vi "subvi voltage to temp to write.vi"(9 "Thermistor 2":T1={"sampling freq: fs 2"=200.0, "low cutoff freq: fl 2"=5.0, "order 2"=3} {"low cutoff freq: fl 2" format="%#_13g"; "sampling freq: fs 2" format="%#_13g"}, 10 "Thermistor 1":T2, 11 "data":dynamicdata(waveform)) -> (0 "Thermistor 1 and 2":cluster{"Filtered x":dbl, "Filtered x":dbl}(graph))   [LabVIEW 2021]
uses:
  <vilib>/express/express shared/ex_Modify Signal Name.vi
  <vilib>/express/express arith-compare/Formula/XNode/ExpressFormulaBlockNode.xnode
  <vilib>/ptbypt/NI_PtbyPt.lvlib
panel:
  out "Thermistor 2 Filtered":dbl(graph)
  out "Thermistor 2 Unfiltered":waveform(dbl)(graph)
  out "Thermistor 1 Filtered":dbl(graph)
  out "Thermistor 1 Unfiltered":waveform(dbl)(graph)
  out "Waveform Chart":dynamicdata(graph)
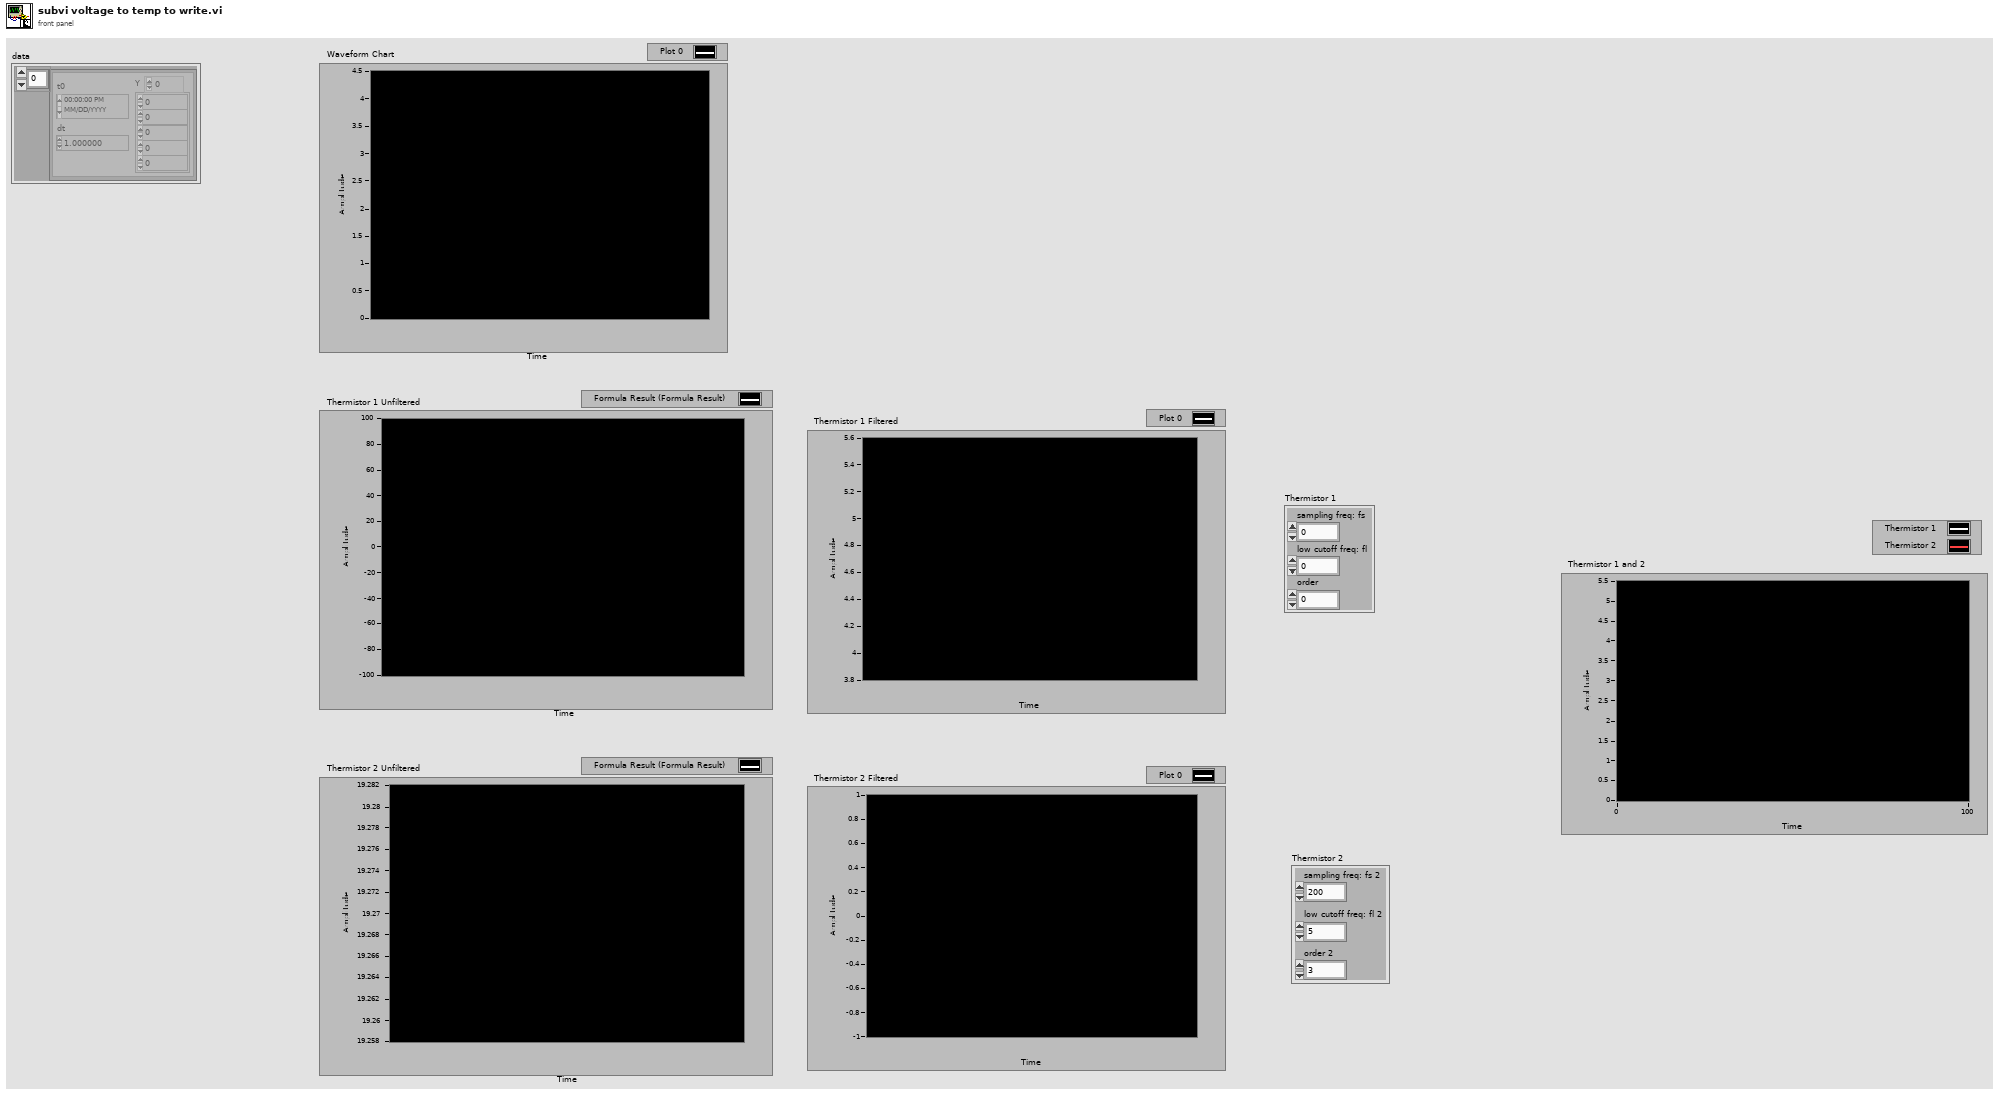
[diagram p1: front panel]
types:
  T1 = cluster{"sampling freq: fs 2":dbl, "low cutoff freq: fl 2":dbl, "order 2":i32}
  T2 = cluster{"sampling freq: fs":dbl, "low cutoff freq: fl":dbl, "order":i32}
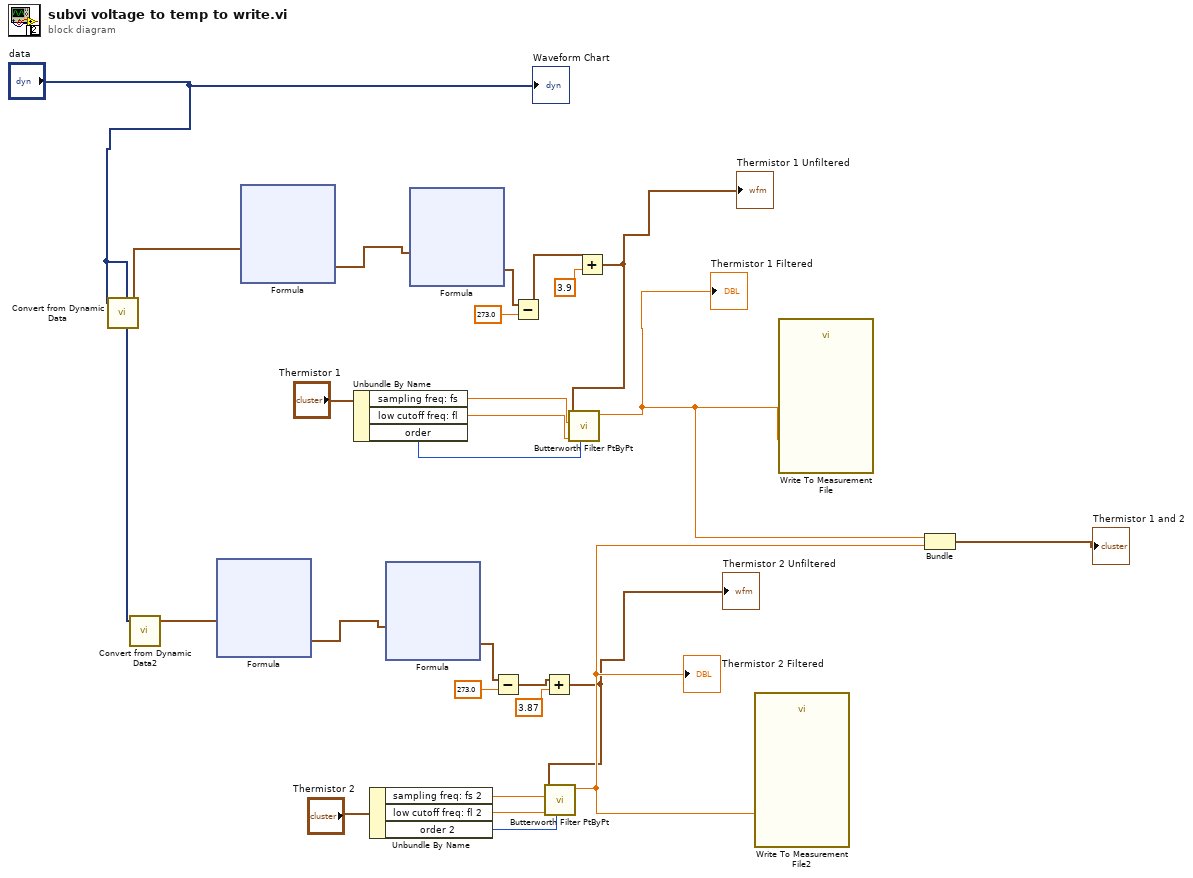
[diagram p0: block diagram]
diagram:
  n1 = call "Convert from Dynamic Data"("Dynamic Data Type"="data") -> ("Waveform"=w26:waveform(dbl))  [unwired: 3 in]
  n2 = call "Convert from Dynamic Data2"("Dynamic Data Type"="data") -> ("Waveform"=w20:waveform(dbl))  [unwired: 3 in]
  n3 = xnode "Formula"("v"=w20) -> ("Result"=w21:waveform(dbl))  [unwired: 1 in, 1 out]
  n4 = xnode "Formula"("v"=w26) -> ("Result"=w24:waveform(dbl))  [unwired: 1 in, 1 out]
  n5 = Unbundle By Name("Thermistor 1") -> ("sampling freq: fs"=w14:dbl, "low cutoff freq: fl"=w13:dbl, "order"=w12:i32)
  n6 = Unbundle By Name("Thermistor 2") -> ("sampling freq: fs 2"=w10:dbl, "low cutoff freq: fl 2"=w9:dbl, "order 2"=w8:i32)
  n7 = xnode "Formula"("R"=w21) -> ("Result"=w22:waveform(dbl))  [unwired: 1 in, 1 out]
  n8 = xnode "Formula"("R"=w24) -> ("Result"=w6:waveform(dbl))  [unwired: 1 in, 1 out]
  n9 = Subtract(x=w22, y=273.0) -> (x-y=w2:waveform(dbl))
  n10 = Subtract(x=w6, y=273.0) -> (x-y=w5:waveform(dbl))
  n11 = Add(x=w2, y=3.87) -> (x+y=w1:waveform(dbl))
  "Thermistor 2 Unfiltered" <- w1
  n12 = call <vilib>:"Butterworth Filter PtByPt.vi"("order"=w8, "low cutoff freq: fl"=w9, "sampling freq: fs"=w10, "x"=w1) -> ("Filtered x"=w17:dbl)  [unwired: 5 in, 1 out]
  "Thermistor 2 Filtered" <- w17
  n13 = Add(x=w5, y=3.9) -> (x+y=w4:waveform(dbl))
  "Thermistor 1 Unfiltered" <- w4
  n14 = call <vilib>:"Butterworth Filter PtByPt.vi"("order"=w12, "low cutoff freq: fl"=w13, "sampling freq: fs"=w14, "x"=w4) -> ("Filtered x"=w18:dbl)  [unwired: 5 in, 1 out]
  "Thermistor 1 Filtered" <- w18
  n15 = call "Write To Measurement File2"("Signals"=w17) -> ()  [unwired: 16 in, 3 out]
  n16 = call "Write To Measurement File"("Signals"=w18) -> ()  [unwired: 16 in, 3 out]
  n17 = Bundle("Filtered x"=w18, "Filtered x"=w17) -> (→"Thermistor 1 and 2":cluster{"Filtered x":dbl, "Filtered x":dbl})  [unwired: 1 in]
  "Waveform Chart" <- "data"
